vi "Ref Memory.vi"(7 "Operation":T1, 8 "error in":errorcluster, 10 "Name In":string, 11 "Ref In":refnum<vi>) -> (0 "error out":errorcluster, 2 "Name Out":string, 3 "Ref Out":refnum<vi>)   [LabVIEW 2012]
uses:
  Controls/Ref Memory Operations.ctl
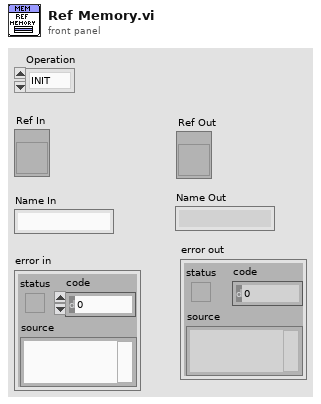
[diagram p1: front panel]
types:
  T1 = typedef "Ref Memory Operations.ctl" = enum16{"INIT", "WRITE", "READ"}
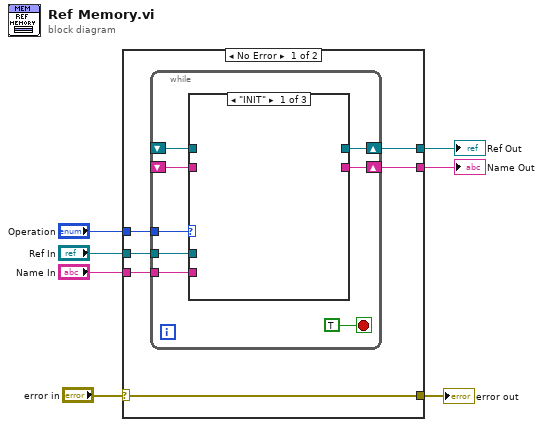
[diagram p0: block diagram]
diagram:
  n1 = case shown="No Error" "error in" {
    selector: "error in" -> [w8 w26]
    tunnel: "Ref In" -> [w13 _]
    tunnel: "Name In" -> [w12 _]
    tunnel: "Operation" -> [w11 _]
    tunnel: [w10 _] -> w4
    tunnel: [w9 _] -> w3
    tunnel: [w8 w26] -> w1
    frame No Error {
      n2 = while {
        tunnel: w13 -> [w18]
        tunnel: w12 -> [w16]
        tunnel: w11 -> [w20]
        shift-right: [w19] -> w10
        shift-left: _ -> [w15]
        shift-right: [w17] -> w9
        shift-left: _ -> [w14]
        stop <- TRUE stop-if-true
        n3 = case shown="\"INIT\"" w20 {
          tunnel: [_ w23 w25] -> w19
          tunnel: w18 -> [_ w23 _]
          tunnel: [_ w22 w24] -> w17
          tunnel: w16 -> [_ w22 _]
          tunnel: w15 -> [_ _ w25]
          tunnel: w14 -> [_ _ w24]
          frame "INIT" {
          }
          frame "WRITE" {
          }
          frame "READ" {
          }
        }
      }
    }
    frame Error {
    }
  }
  "Ref Out" <- w4
  "Name Out" <- w3
  "error out" <- w1
